vi "Check Change Result.vi"(8 "error in (no error)":errorcluster, 9 "Old Val":T4, 10 "New Val":T4, 11 "GroupLoggingControl in":refnum<class "GroupLoggingControl.lvclass">) -> (0 "error out":errorcluster, 1 "Node (Empty = All)":string, 2 "Log Group":T1, 3 "GroupLoggingControl out":refnum<class "GroupLoggingControl.lvclass">)   [LabVIEW 2020, in "VolatusGUIElements.lvlib" / "GroupLoggingControl.lvclass"]
uses:
  GroupLoggingControl.lvclass
  Log Group.ctl
  Log Group Status.ctl
  Command Info.ctl
  GroupLoggingControl.lvclass/GroupLoggingControl.ctl
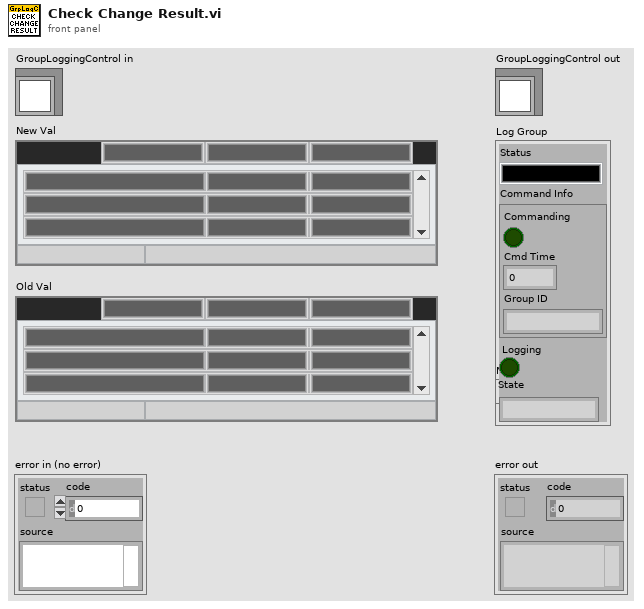
[diagram p1: front panel]
types:
  T1 = typedef "VolatusGUIElements.lvlib/GroupLoggingControl.lvclass/Log Group.ctl" = cluster{"Status":T2, "Command Info":T3, "Logging":bool, "State":string}
  T2 = typedef "VolatusGUIElements.lvlib/GroupLoggingControl.lvclass/Log Group Status.ctl" = cluster{"Group":string, "Group Color":u32, "Button":bool}
  T3 = typedef "VolatusGUIElements.lvlib/GroupLoggingControl.lvclass/Command Info.ctl" = cluster{"Commanding":bool, "Cmd Time":dbl, "Group ID":string}
  T4 = cluster{"Series":string, "Timestamp":string, "Targets":cluster{"Node":string, "Node Color":u32, "Groups":cluster{"Group":string, "Group Color":u32, "Button":bool}[]}[], "Groups":cluster{"Group":string, "Group Color":u32, "Button":bool}[]}
  T5 = typedef "VolatusGUIElements.lvlib/GroupLoggingControl.lvclass/Status.ctl" = cluster{"Groups":T1[], "Targets":T6[]}
  T6 = typedef "VolatusGUIElements.lvlib/GroupLoggingControl.lvclass/Target Info.ctl" = cluster{"Node":string, "Node Color":u32, "Groups":T1[]}
  T7 = cluster{"Series":bool, "Timestamp":bool, "Targets":cluster{"Node":bool, "Node Color":bool, "Groups":cluster{"Group":bool, "Group Color":bool, "Button":bool}[]}[], "Groups":cluster{"Group":bool, "Group Color":bool, "Button":bool}[]}
  T8 = cluster{"Node":bool, "Node Color":bool, "Groups":cluster{"Group":bool, "Group Color":bool, "Button":bool}[]}[]
  T9 = cluster{"Group":bool, "Group Color":bool, "Button":bool}[]
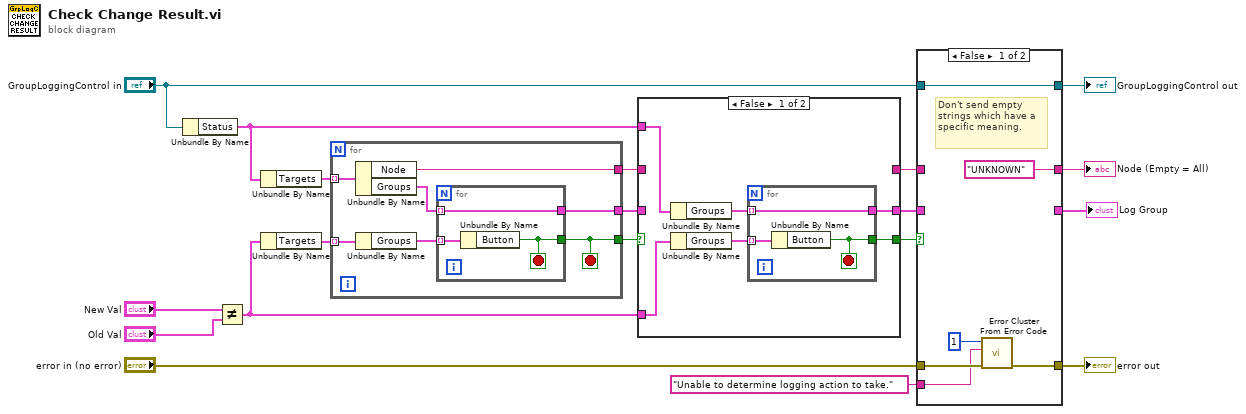
[diagram p0: block diagram]
diagram:
  n1 = Unbundle By Name("GroupLoggingControl in") -> ("Status"=w12:T5)
  n2 = Not Equal?(x="New Val", y="Old Val") -> (x != y?=w11:T7)
  n3 = Unbundle By Name(w12) -> ("Targets"=w16:T6[])
  n4 = Unbundle By Name(w11) -> ("Targets"=w18:T8)
  n5 = for {
    tunnel: w18 -> [w26] mode=indexing
    tunnel: w16 -> [w24] mode=indexing
    tunnel: [w22] -> w13
    tunnel: [w21] -> w14
    tunnel: [w20] -> w15
    stop <- w20 stop-if-true
    n6 = Unbundle By Name(w24) -> ("Node"=w22:string, "Groups"=w23:T1[])
    n7 = Unbundle By Name(w26) -> ("Groups"=w25:T9)
    n8 = for {
      tunnel: w25 -> [w29] mode=indexing
      tunnel: w23 -> [w27] mode=indexing
      tunnel: [w27] -> w21
      tunnel: [w28] -> w20
      stop <- w28 stop-if-true
      n9 = Unbundle By Name(w29) -> ("Button"=w28:bool)
    }
  }
  n10 = case shown="False" w15 {
    selector: w15 -> [_ w39]
    tunnel: w14 -> [_ w40]
    tunnel: w13 -> [_ w41]
    tunnel: [_ w41] -> w9
    tunnel: [w31 w40] -> w8
    tunnel: w12 -> [w35 _]
    tunnel: w11 -> [w34 _]
    tunnel: [w30 w39] -> w10
    frame False {
      n11 = Unbundle By Name(w35) -> ("Groups"=w32:T1[])
      n12 = Unbundle By Name(w34) -> ("Groups"=w33:T9)
      n13 = for {
        tunnel: w33 -> [w38] mode=indexing
        tunnel: w32 -> [w36] mode=indexing
        tunnel: [w36] -> w31
        tunnel: [w37] -> w30
        stop <- w37 stop-if-true
        n14 = Unbundle By Name(w38) -> ("Button"=w37:bool)
      }
    }
    frame True {
      # "Target specific Group command"
    }
  }
  n15 = case shown="False" w10 {
    tunnel: w9 -> [_ w51]
    tunnel: w8 -> [_ w50]
    tunnel: ["UNKNOWN" ("Node") w51] -> w7
    tunnel: [_ w50] -> w1
    tunnel: "GroupLoggingControl in" -> [w47 w49]
    tunnel: [w47 w49] -> w5
    tunnel: "error in (no error)" -> [w45 w48]
    tunnel: [w44 w48] -> w3
    tunnel: "Unable to determine logging action to take." -> [w42 _]
    frame False {
      # "Don't send empty strings which have a specific meaning."
      n16 = call <vilib>:"Error Cluster From Error Code.vi"("error in (no error)"=w45, "error message (\"\")"=w42, "error code (0)"=1) -> ("error out"=w44:errorcluster)  [unwired: 6 in]
    }
    frame True {
    }
  }
  "error out" <- w3
  "GroupLoggingControl out" <- w5
  "Node (Empty = All)" <- w7
  "Log Group" <- w1
